vi "test-Coordinate-System-ALL-TESTS.vi"(8 "error in (no error)":errorcluster) -> (0 "error out":errorcluster, 3 "All Passed":bool)   [LabVIEW 2019]
panel:
  out "Test 6":bool
  out "Test 5":bool
  out "Test 4":bool
  out "Test 3":bool
  out "Test 2":bool
  out "Test 1":bool
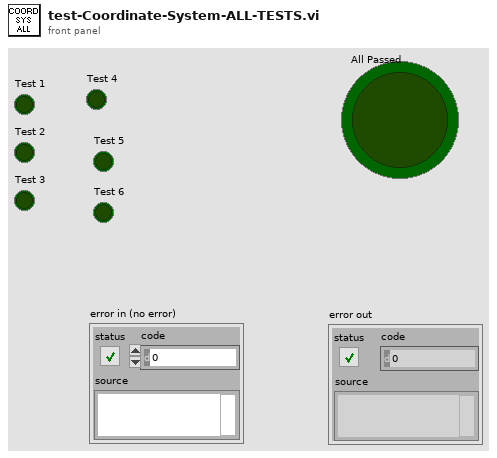
[diagram p1: front panel]
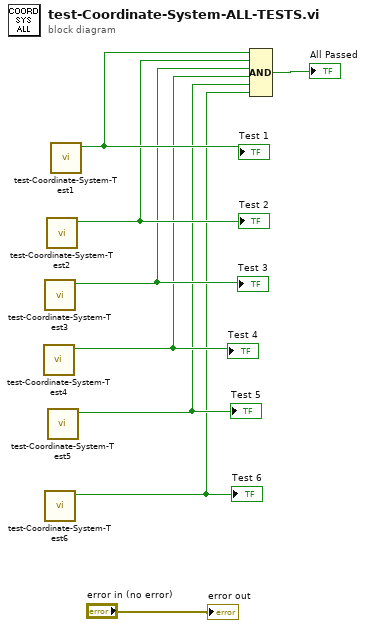
[diagram p0: block diagram]
diagram:
  n1 = call "test-Coordinate-System-Test4.vi"() -> ("All tests passed"=w3:bool)  [unwired: 11 in]
  "Test 4" <- w3
  n2 = call "test-Coordinate-System-Test3.vi"() -> ("All tests passed"=w4:bool)  [unwired: 11 in]
  "Test 3" <- w4
  n3 = call "test-Coordinate-System-Test6.vi"() -> ("All tests passed"=w1:bool)  [unwired: 11 in]
  "Test 6" <- w1
  n4 = call "test-Coordinate-System-Test2.vi"() -> ("All tests passed"=w5:bool)  [unwired: 11 in]
  "Test 2" <- w5
  n5 = call "test-Coordinate-System-Test5.vi"() -> ("All tests passed"=w2:bool)  [unwired: 11 in]
  "Test 5" <- w2
  n6 = call "test-Coordinate-System-Test1.vi"() -> ("All tests passed"=w6:bool)  [unwired: 11 in]
  "Test 1" <- w6
  n7 = Compound Arithmetic op=AND(w6, w5, w4, w3, w2, w1) -> (→"All Passed":bool)
  "error out" <- "error in (no error)"
